vi "Create WS Client.vi"(8 "error in (no error)":errorcluster, 9 "TCP":refnum<k5>, 10 "Request":refnum<class "Request.lvclass">, 11 "Basic WebSocket Manager in":refnum<class "Basic WebSocket Manager.lvclass">) -> (0 "error out":errorcluster, 2 "WS Client":refnum<class "WebSocket Client.lvclass">)   [LabVIEW 2020, in "HTTP Server.lvlib" / "Basic WebSocket Manager.lvclass"]
uses:
  Basic WebSocket Manager.lvclass
  lv-http-util/HTTP Utils/Request/Request.lvclass
  WebSocket Client/WebSocket Client.lvclass
  Basic WebSocket Manager.lvclass/Basic WebSocket Manager.ctl
  lv-promises/Promises/Promise/Promise.lvclass
  Create Client Data.ctl
  lv-promises/Promises/Future/Future.lvclass
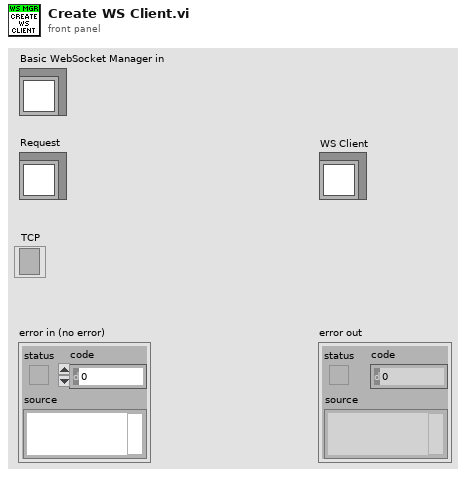
[diagram p1: front panel]
types:
  T1 = typedef "HTTP Server.lvlib/Basic WebSocket Manager.lvclass/Create Client Data.ctl" = cluster{"Request":refnum<class "Request.lvclass">, "TCP":refnum<k5>, "Promise":refnum<class "Promise.lvclass">}
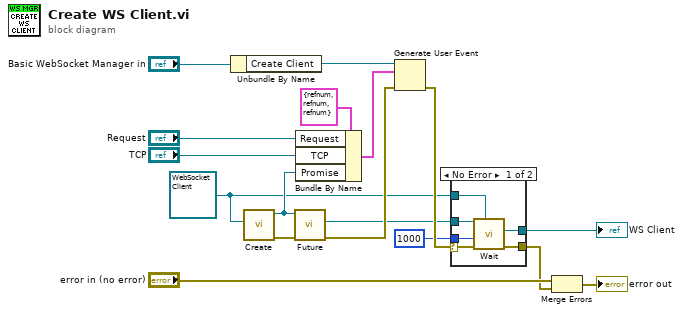
[diagram p0: block diagram]
diagram:
  w8 = refnum<class "WebSocket Client.lvclass"> refnum ("HTTP Server:WebSocket Client.lvclass")
  n1 = Unbundle By Name("Basic WebSocket Manager in") -> ("Create Client"=w6:refnum<user-event>)
  n2 = call "Create.vi"("Result Type (None)"=w8) -> ("error out"=w15:errorcluster, "Promise"=w12:refnum<class "Promise.lvclass">)  [unwired: 9 in]
  n3 = call "Future.vi"("Promise in"=w12) -> ("Future"=w9:refnum<class "Future.lvclass">)  [unwired: 9 in, 1 out]
  n4 = Bundle By Name(cluster=T1 {"Request"=refnum, "TCP"=refnum, "Promise"=refnum} ("Create Client Data"), "Request"="Request", "TCP"="TCP", "Promise"=w12) -> (w5:T1)
  n5 = Generate User Event(user event=w6, event data cluster=w5, error in=w15) -> (error out=w16:errorcluster)  [unwired: 1 in, 1 out]
  n6 = case shown="No Error" w16 {
    selector: w16 -> [w20 w23]
    tunnel: w9 -> [w22 _]
    tunnel: w8 -> [w21 _]
    tunnel: [w19 _] -> w4
    tunnel: [w18 w23] -> w2
    tunnel: 1000 ("Timeout mS (-1)") -> [w17 _]
    frame No Error {
      n7 = call "Wait.vi"("Result Type"=w21, "error in (no error)"=w20, "Timeout mS (-1)"=w17, "Future in"=w22) -> ("error out"=w18:errorcluster, "Result"=w19:refnum<class "WebSocket Client.lvclass">)  [unwired: 6 in]
    }
    frame Error {
    }
  }
  "WS Client" <- w4
  n8 = Merge Errors("error in (no error)", w2) -> (→"error out":errorcluster)
